vi "ttm_tensile_poller.vi"   [LabVIEW 2011]
types:
  T1 = cluster{"Name":string, "Type":i32, "SI Full Scale":dbl, "Full Scale":dbl, "Units String":string, "Display Format":string, "Gauge Length":dbl}[][]
  T2 = cluster{"Device ID":i32, "Device Name":string, "Device Type":i32}[]
  T3 = cluster{"Set Point Time":dbl, "Set Point Time":dbl, "Double":dbl, "Double":dbl}
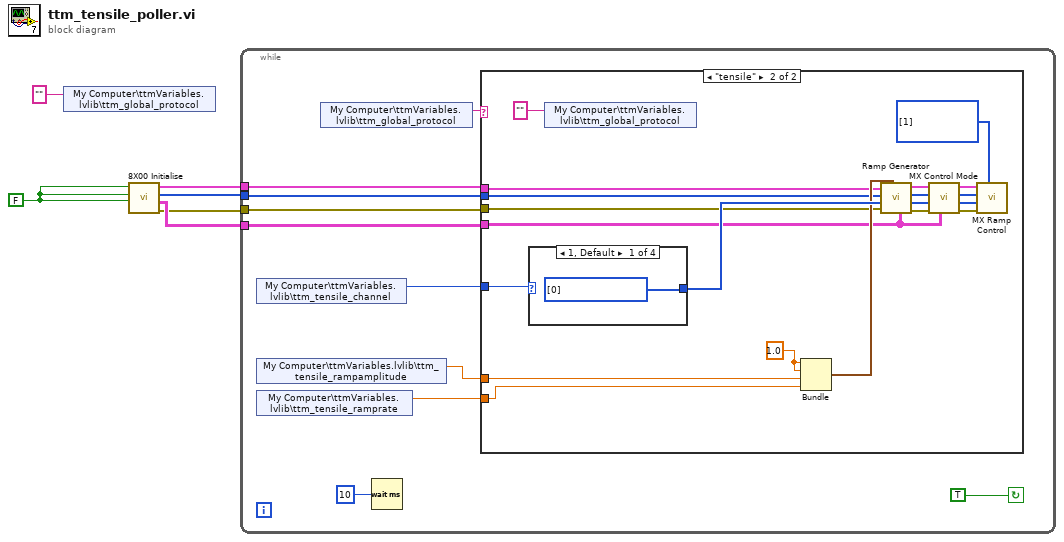
[diagram p0: block diagram]
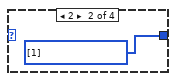
[diagram p3: hidden frame]
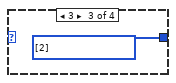
[diagram p4: hidden frame]
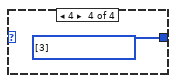
[diagram p5: hidden frame]
diagram:
  w2 = FALSE ("Reset?")
  n1 = shared-variable "My Computer\\ttmVariables.lvlib\\ttm_global_protocol"("" ("protocol")) -> ()  [unwired: 1 in, 1 out]
  n2 = call "8X00 Initialise.vi"("Reset?"=w2, "Create DVM? (T)"=w2, "Create Console? (T)"=w2) -> ("error out"=w3:errorcluster, "Channel Data"=w6:T1, "Axis Selector"=w4:i32[], "Axis Information"=w5:T2)  [unwired: 1 in]
  n3 = while {
    tunnel: w6 -> [w13]
    tunnel: w5 -> [w14]
    tunnel: w4 -> [w15]
    tunnel: w3 -> [w12]
    stop <- TRUE continue-if-true
    n4 = shared-variable "My Computer\\ttmVariables.lvlib\\ttm_tensile_channel"() -> (w8:i32)  [unwired: 1 in, 1 out]
    n5 = shared-variable "My Computer\\ttmVariables.lvlib\\ttm_tensile_rampamplitude"() -> (w11:dbl)  [unwired: 1 in, 1 out]
    n6 = shared-variable "My Computer\\ttmVariables.lvlib\\ttm_tensile_ramprate"() -> (w10:dbl)  [unwired: 1 in, 1 out]
    n7 = shared-variable "My Computer\\ttmVariables.lvlib\\ttm_global_protocol"() -> (w7:string)  [unwired: 1 in, 1 out]
    n8 = Wait (ms)(milliseconds to wait=u32 10) -> ()  [unwired: 1 out]
    n9 = case shown="\"tensile\"" w7 {
      tunnel: w15 -> [_ w33]
      tunnel: w14 -> [_ w32]
      tunnel: w13 -> [_ w18]
      tunnel: w12 -> [_ w31]
      tunnel: w11 -> [_ w30]
      tunnel: w10 -> [_ w29]
      tunnel: w8 -> [_ w28]
      frame "", Default {
      }
      frame "tensile" {
        w27 = u16[] [1] items=["Stop", "Start or continue", "Hold", "Continue", "Return ramp to set level at fixed rate", "Reserved", "Reserved", "Start Random without demand hold", "Start Random with demand hold", "Prepare Random Start without demand hold", "Prepare Random Start with demand hold", "Unslave", "Reserved", "Reserved", "Start Sample Data Playback or Resume", "Prepare for Start of Sample Data", "Reserved", "Reserved", "Resume Playback", "Start an electromechanical frame return"] ("Ramp Control")
        w36 = 1.0 ("Set Point Time")
        n10 = case shown="1, Default" w28 {
          tunnel: [w37 w38 w39 w40] -> w35
          frame 1, Default {
            w37 = u16[] [0] items=["Channel 1", "Channel 2", "Channel 3", "Channel 4"] ("Choose channel to apply\nthe setpoint")
          }
          frame 2 {
            w38 = u16[] [1] items=["Channel 1", "Channel 2", "Channel 3", "Channel 4"] ("Choose channel to apply\nthe setpoint")
          }
          frame 3 {
            w39 = u16[] [2] items=["Channel 1", "Channel 2", "Channel 3", "Channel 4"] ("Choose channel to apply\nthe setpoint")
          }
          frame 4 {
            w40 = u16[] [3] items=["Channel 1", "Channel 2", "Channel 3", "Channel 4"] ("Choose channel to apply\nthe setpoint")
          }
        }
        n11 = shared-variable "My Computer\\ttmVariables.lvlib\\ttm_global_protocol"("" ("protocol")) -> ()  [unwired: 1 in, 1 out]
        n12 = Bundle("Set Point Time"=w36, "Set Point Time"=w36, "Double"=w30, "Double"=w29) -> (w34:T3)  [unwired: 1 in]
        n13 = call "Ramp Generator.vi"("Channel Data"=w18, "Input cluster"=w34, "error in (no error)"=w31, "Channels"=w35, "Axis Selector"=w33, "Axis Information"=w32) -> ("Error Out"=w19:errorcluster, "Channels Out"=w20:u16[], "Axis Selector Out"=w21:i32[], "Axis Information Out"=w22:T2)  [unwired: 2 in]
        n14 = call "MX Control Mode.vi"("Channel Data"=w18, "error in (no error)"=w19, "Control Modes"=w20, "Axis Selector"=w21, "Axis Information"=w22) -> ("error out"=w26:errorcluster, "Control Modes out"=w25:u16[], "Axis Selector out"=w24:i32[], "Axis Information out"=w23:T2)  [unwired: 1 in]
        n15 = call "MX Ramp Control.vi"("Ramp Control"=w27, "error in (no error)"=w26, "Channels In"=w25, "Axis Selector In"=w24, "Axis Information In"=w23) -> ()  [unwired: 2 in, 4 out]
      }
    }
  }
